vi "initialise.vi"(8 "error in (no error)":errorcluster, 11 "GenericPlugin in":refnum<class "ComponentTemplate.lvclass">) -> (0 "error out":errorcluster, 3 "GenericPlugin out":refnum<class "ComponentTemplate.lvclass">)   [LabVIEW 2010]
doc: "The dynamic dispatch-version of this VI initalises the plug-in object by allocating and initalising any dynamic resources need."
uses:
  ComponentTemplate.lvclass
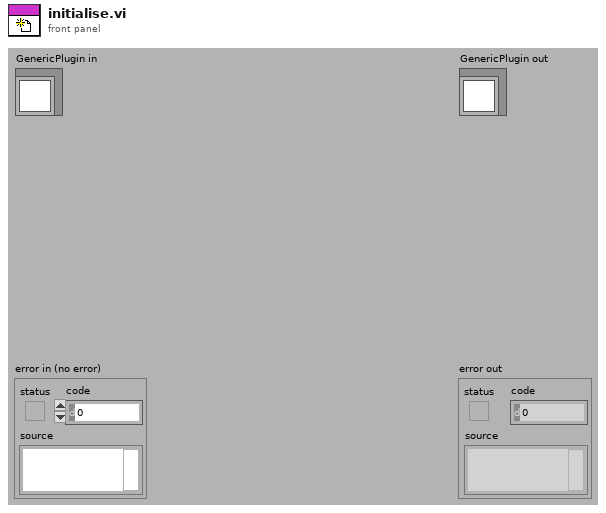
[diagram p1: front panel]
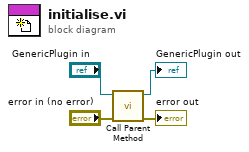
[diagram p0: block diagram]
diagram:
  n1 = call-parent "Call Parent Method"("error in (no error)"="error in (no error)", "GenericPlugin in"="GenericPlugin in") -> ("error out"=→"error out":errorcluster, "GenericPlugin out"=→"GenericPlugin out":refnum<class "ComponentTemplate.lvclass">)  [unwired: 8 in]
